vi "ManualClimb.vi"(10 "CopilotPOV":i16, 11 "CopilotAxes":dbl[](array[numeric])) -> (0 "ActuateBackClimb":dbl, 1 "ActuateFrontClimb":dbl, 2 "DropWheel":bool, 3 "ClimbDrive":bool)   [LabVIEW 2018]
uses:
  Globals.vi
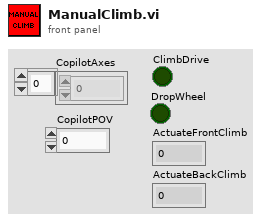
[diagram p1: front panel]
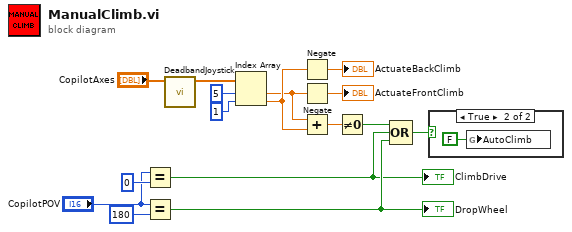
[diagram p0: block diagram]
diagram:
  n1 = Equal?(x="CopilotPOV", y=i16 0) -> (x = y?=w5:bool)
  "ClimbDrive" <- w5
  n2 = Equal?(x="CopilotPOV", y=i16 180) -> (x = y?=w11:bool)
  "DropWheel" <- w11
  n3 = call "DeadbandJoystick.vi"("InputArray"="CopilotAxes") -> ("OutputArray"=w7:dbl[])  [unwired: 10 in]
  n4 = Index Array(array=w7, index #1=5 ("index"), index #2=1 ("index")) -> (element #1=w4:dbl, element #2=w6:dbl)
  n5 = Negate(x=w6) -> (-x=→"ActuateBackClimb":dbl)
  n6 = Negate(x=w4) -> (-x=→"ActuateFrontClimb":dbl)
  n7 = Add(x=w4, y=w6) -> (x+y=w13:dbl)
  n8 = Not Equal To 0?(x=w13) -> (x != 0?=w3:bool)
  n9 = Compound Arithmetic op=OR(w3, w5, w11) -> (w9:bool)
  n10 = case shown="True" w9 {
    frame False {
    }
    frame True {
      n11 = global write "Globals.vi" "AutoClimb"(FALSE ("AutoClimb")) -> ()
    }
  }
